vi "Sort Offspring In Ascending Order.vi"(11 "OffSpring":T1[](array[typedef])) -> (2 "Offspring In Ascending Fitness Order":T1[](array[typedef]), 3 "Fitness Values In Ascending Order":u16[](array[numeric]))   [LabVIEW 2013, in "GA.lvclass"]
uses:
  GA.lvclass
  Controls/Solution_GA.ctl
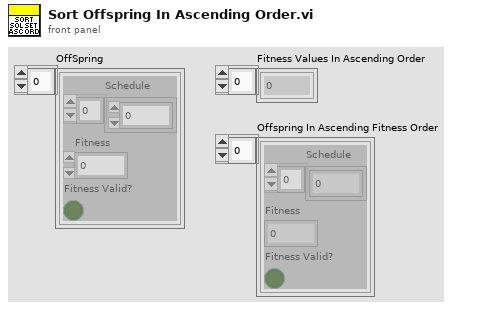
[diagram p1: front panel]
types:
  T1 = typedef "Solution_GA.ctl" = cluster{"Schedule":u16[], "Fitness":u16, "Fitness Valid?":bool}
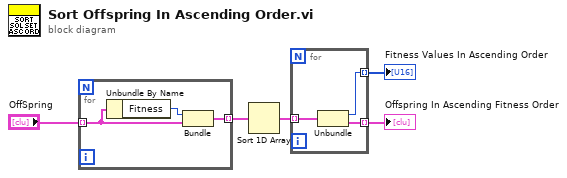
[diagram p0: block diagram]
diagram:
  n1 = for {
    tunnel: [w8] -> w2 mode=indexing
    tunnel: "OffSpring" -> [w7] mode=indexing
    n2 = Unbundle By Name(w7) -> ("Fitness"=w6:u16)
    n3 = Bundle("Fitness"=w6, "Solution"=w7) -> (w8:cluster{"Fitness":u16, "Solution":T1})  [unwired: 1 in]
  }
  n4 = Sort 1D Array(array=w2) -> (sorted array=w1:cluster{"Fitness":u16, "Solution":T1}[])
  n5 = for {
    tunnel: [w11] -> w4 mode=indexing
    tunnel: [w10] -> w3 mode=indexing
    tunnel: w1 -> [w9] mode=indexing
    n6 = Unbundle(w9) -> ("Fitness"=w10:u16, "Solution"=w11:T1)
  }
  "Offspring In Ascending Fitness Order" <- w4
  "Fitness Values In Ascending Order" <- w3
